vi "Delete All Contructors.vi"   [LabVIEW 2015]
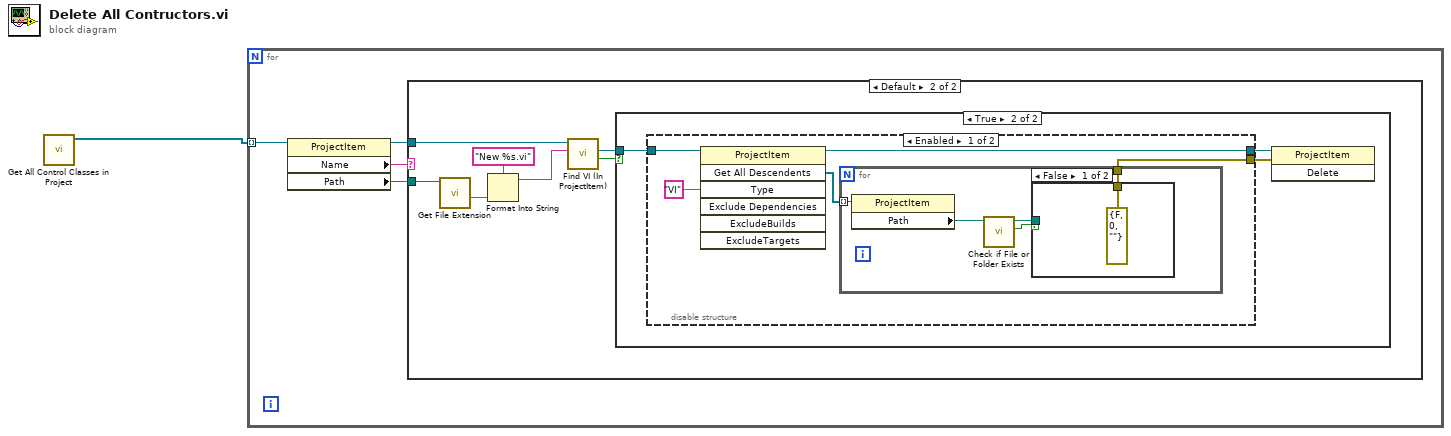
[diagram p0: block diagram]
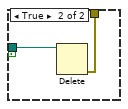
[diagram p4: hidden frame]
diagram:
  n1 = call "Get All Control Classes in Project.vi"() -> ("All Control Classes"=w1:refnum<vi>[])  [unwired: 11 in]
  n2 = for {
    tunnel: w1 -> [w5] mode=indexing
    n3 = property class="ProjectItem"(reference=w5) -> (reference out=w3:refnum<vi>, "Name"=w4:string, "Path"=w2:path)  [unwired: 1 in, 1 out]
    n4 = case shown="Default" w4 {
      tunnel: w3 -> [_ w11]
      tunnel: w2 -> [_ w12]
      frame "Control.lvclass", "GObject.lvclass", "Generic.lvclass" {
      }
      frame Default {
        n5 = call <vilib>:"Get File Extension.vi"("file"=w12) -> ("filename without extension"=w10:string)  [unwired: 6 in, 4 out]
        n6 = Format Into String(format string="New %s.vi", w10) -> (resulting string=w7:string)  [unwired: 2 in, 1 out]
        n7 = call "Find VI (In ProjectItem).vi"("VI Name"=w7, "ProjectItem in"=w11) -> ("Found?"=w6:bool, "VI ProjectItem Refnum"=w9:refnum<vi>)  [unwired: 7 in, 1 out]
        n8 = case shown="True" w6 {
          tunnel: w9 -> [_ w15]
          frame False {
          }
          frame True {
            n9 = disable-structure shown="Enabled" {
              disable-tunnel: w15 -> [w20 w29]
              disable-tunnel: [w19 w29] -> w14
              disable-tunnel: [w18 _] -> w13
              frame Enabled {
                n10 = invoke class="ProjectItem" method="Get All Descendents"(reference=w20, "Type"="VI") -> (reference out=w19:refnum<vi>, "All Descendents"=w17:refnum<vi>[])  [unwired: 5 in, 5 out]
                n11 = for {
                  tunnel: w17 -> [w25] mode=indexing
                  tunnel: [w24] -> w18
                  n12 = property class="ProjectItem"(reference=w25) -> ("Path"=w23:path)  [unwired: 1 in, 2 out]
                  n13 = call <vilib>:"Check if File or Folder Exists.vi"("path"=w23) -> ("file or folder exists?"=w21:bool, "dup path"=w22:path)  [unwired: 8 in, 1 out]
                  n14 = case shown="False" w21 {
                    tunnel: [errorcluster {"status"=FALSE, "code"=0, "source"=""} ("error out") w28] -> w24
                    tunnel: w22 -> [_ w27]
                    frame False {
                    }
                    frame True {
                      n15 = Delete(path (use dialog)=w27) -> (error out=w28:errorcluster)  [unwired: 4 in, 2 out]
                    }
                  }
                }
              }
              frame Disabled {
              }
            }
            n16 = invoke class="ProjectItem" method="Delete"(reference=w14, error in=w13) -> ()  [unwired: 1 in, 3 out]
          }
        }
      }
    }
  }
